vi "Agilent ESG_Close.vi"(8 "error in":errorcluster {"code" format="%.0x"}, 11 "Handle":variant) -> (0 "error out":errorcluster {"code" format="%.0x"})   [LabVIEW 2015]
uses:
  <instrlib>/Agilent ESG Series/Agilent ESG Series.lvlib
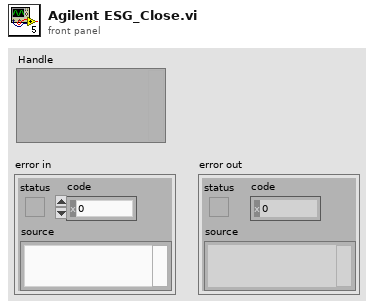
[diagram p1: front panel]
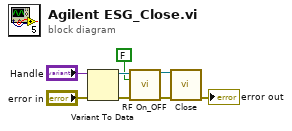
[diagram p0: block diagram]
diagram:
  n1 = Variant To Data(error in="error in", Variant="Handle") -> (data=w5:refnum<visa-resource-name>, error out=w2:errorcluster)  [unwired: 1 in]
  n2 = call <instrlib>:"RF On_OFF.vi"("VISA Resource Name"=w5, "Status (T:ON)"=FALSE, "error in (no error)"=w2) -> ("VISA Resource Name Out"=w4:refnum<visa-resource-name>, "error out"=w3:errorcluster)  [unwired: 11 in]
  n3 = call <instrlib>:"Close.vi"("VISA Resource Name"=w4, "error in (no error)"=w3) -> ("error out"=→"error out":errorcluster)  [unwired: 13 in]
